vi "Format Image Information.vi"(8 "Shutters":T1, 11 "Image Acquisition Parameters":T2={"Scan Type"=enum."Sample Scanning", "Scan Mode"=enum."XY", "Fast Axis Frequency (Hz)"=100.0, "Image Format"=128, "Line Accumulations"=1, "Frames Per Capture"=1, "Frames Accumulations"=1, "Image Dimension (um)"=[], "Number of Z Steps"=1, "Z Steps Size (um)"=1.0, "Pixel Size (nm)"=[], "Customized Image Format"=[]} {"Z Steps Size (um)" min=0.0; "Number of Z Steps" min=1; "Frames Accumulations" min=1; "Frames Per Capture" min=1; "Line Accumulations" min=1; "Image Format" items=["64 x 64"=64, "128 x 128"=128, "256 x 256"=256, "512 x 512"=512, "1024 x 1024"=1024, "2048 x 2048"=2048, "Customized..."=0]}) -> (2 "Result":string)   [LabVIEW 2014]
uses:
  Type Defs/Image Acquisition Parameters.ctl
panel:
  # "Length"
  # "Height"
  # "XY"
  # "Z"
  # "Length"
  # "Height"
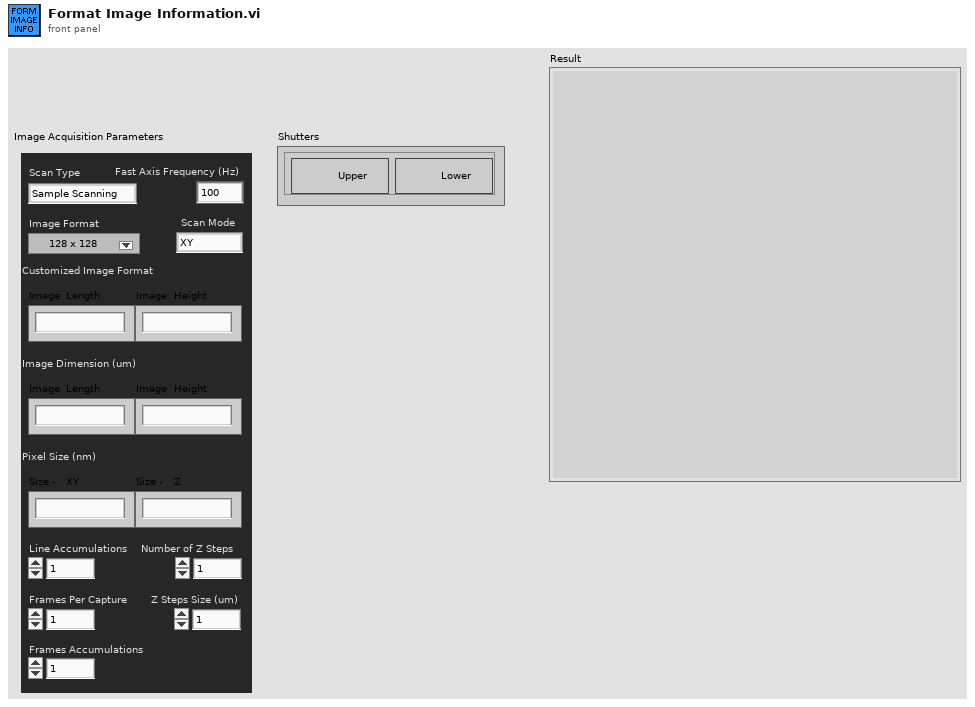
[diagram p1: front panel]
types:
  T1 = cluster{"Upper Shutter":bool, "Lower Shutter":bool}
  T2 = typedef "Image Acquisition Parameters.ctl" = cluster{"Scan Type":enum16{"Sample Scanning", "Beam Scanning"}, "Scan Mode":enum16{"XY", "XZ", "YZ", "XYZ"}, "Fast Axis Frequency (Hz)":dbl, "Image Format":u16, "Line Accumulations":u16, "Frames Per Capture":u16, "Frames Accumulations":u16, "Image Dimension (um)":dbl[], "Number of Z Steps":u16, "Z Steps Size (um)":dbl, "Pixel Size (nm)":dbl[], "Customized Image Format":dbl[]}
  T3 = typedef "Laser Controls.ctl" = cluster{"STED Power (V)":dbl, "STED":bool, "650 nm":bool, "590 nm":bool, "485 nm":bool, "Manual Control":bool}
  T4 = typedef "Detectors.ctl" = cluster{"PMT":bool, "Far Red (685/40 nm)":bool, "Orange (624/40 nm)":bool, "Green (525/50 nm)":bool, "Sum All":bool}
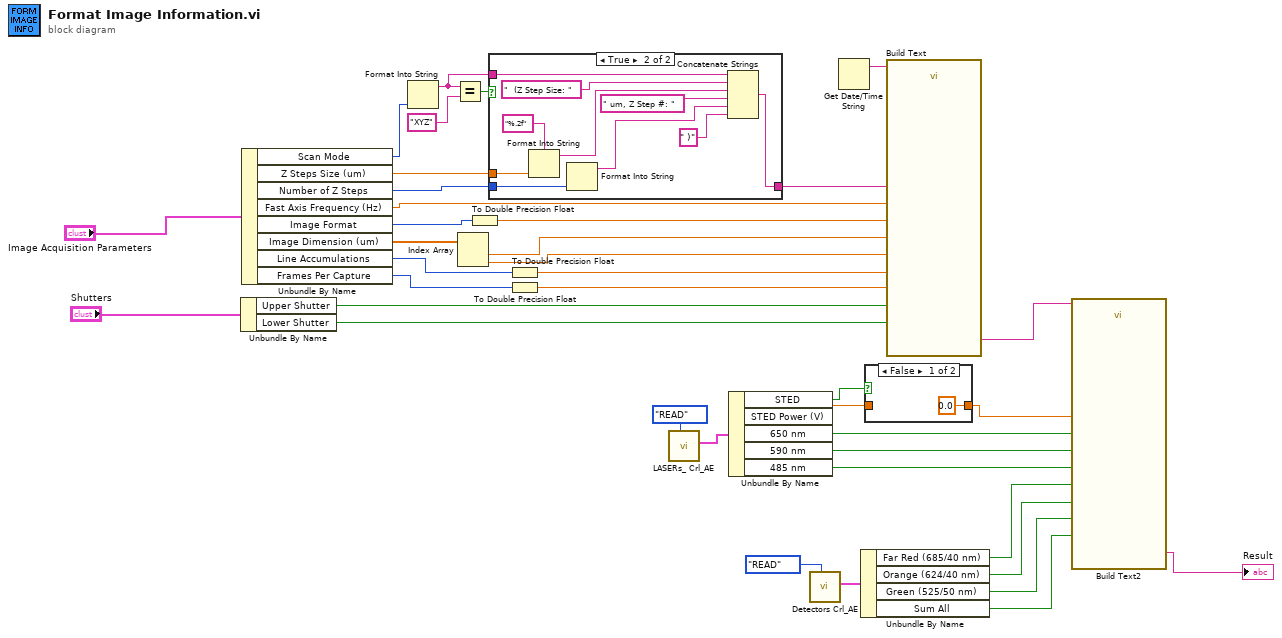
[diagram p0: block diagram]
diagram:
  n1 = Unbundle By Name("Shutters") -> ("Upper Shutter"=w15:bool, "Lower Shutter"=w14:bool)
  n2 = Unbundle By Name("Image Acquisition Parameters") -> ("Scan Mode"=w3:enum16{"XY", "XZ", "YZ", "XYZ"}, "Z Steps Size (um)"=w2:dbl, "Number of Z Steps"=w1:u16, "Fast Axis Frequency (Hz)"=w36:dbl, "Image Format"=w35:u16, "Image Dimension (um)"=w37:dbl[], "Line Accumulations"=w34:u16, "Frames Per Capture"=w33:u16)
  n3 = Format Into String(w3) -> (resulting string=w4:string)  [unwired: 3 in, 1 out]
  n4 = Equal?(x=w4, y="XYZ") -> (x = y?=w5:bool)
  n5 = Index Array(array=w37) -> (element #1=w11:dbl, element #2=w10:dbl)  [unwired: 2 in]
  n6 = To Double Precision Float(number=w35) -> (double precision float=w12:dbl)
  n7 = case shown="True" w5 {
    tunnel: [w39 w47] -> w7
    tunnel: w4 -> [w39 w49]
    tunnel: w2 -> [_ w46]
    tunnel: w1 -> [_ w42]
    frame False {
    }
    frame True {
      n8 = Format Into String(format string="%.2f", w46) -> (resulting string=w45:string)  [unwired: 2 in, 1 out]
      n9 = Format Into String(w42) -> (resulting string=w41:string)  [unwired: 3 in, 1 out]
      n10 = Concatenate Strings(w49, "  (Z Step Size: " ("string"), w45, " um, Z Step #: " ("string"), w41, " )" ("string")) -> (w47:string)
    }
  }
  n11 = To Double Precision Float(number=w34) -> (double precision float=w9:dbl)
  n12 = To Double Precision Float(number=w33) -> (double precision float=w8:dbl)
  n13 = call "LASERs_ Crl_AE.vi"("Action"=enum16{"READ", "WRITE"}."READ") -> ("Laser Parameters Out"=w32:T3)  [unwired: 10 in]
  n14 = Unbundle By Name(w32) -> ("STED"=w30:bool, "STED Power (V)"=w29:dbl, "650 nm"=w27:bool, "590 nm"=w18:bool, "485 nm"=w26:bool)
  n15 = call "Detectors Crl_AE.vi"("Action"=enum16{"READ", "WRITE"}."READ") -> ("Detectors Parameters Out"=w23:T4)  [unwired: 10 in]
  n16 = Get Date/Time String() -> (date string=w16:string)  [unwired: 3 in, 1 out]
  n17 = Unbundle By Name(w23) -> ("Far Red (685/40 nm)"=w22:bool, "Orange (624/40 nm)"=w21:bool, "Green (525/50 nm)"=w20:bool, "Sum All"=w19:bool)
  n18 = case shown="False" w30 {
    tunnel: w29 -> [_ w51]
    tunnel: [0.0 ("STED Power (V)") w51] -> w28
    frame False {
    }
    frame True {
    }
  }
  n19 = call "Build Text"("Beginning Text"=w16, "Scan Mode:"=w7, "Fast Axis Frequency (Hz)"=w36, "Image Format:"=w12, "Image Height:"=w10, "Image Width:"=w11, "Line Accumulations:"=w9, "Number of Frames:"=w8, "Upper Shutter"=w14, "Lower Shutter"=w15) -> ("Result"=w13:string)  [unwired: 16 in, 1 out]
  n20 = call "Build Text2"("Beginning Text"=w13, "485 laser"=w26, "Orange (624/40 nm)"=w21, "Sum All detectors"=w19, "STED Power (V)"=w28, "650 laser"=w27, "590 laser"=w18, "Far Red (697/75 nm)"=w22, "Green(525/50nm)"=w20) -> ("Result"=→"Result":string)  [unwired: 5 in, 1 out]
